vi "Send Value.vi"(8 "error in":errorcluster, 11 "Value":dbl) -> (0 "error out":errorcluster)   [LabVIEW 2014, in "Chart Module.lvlib"]
uses:
  Chart Module.lvlib
  Send Value Argument--cluster.ctl
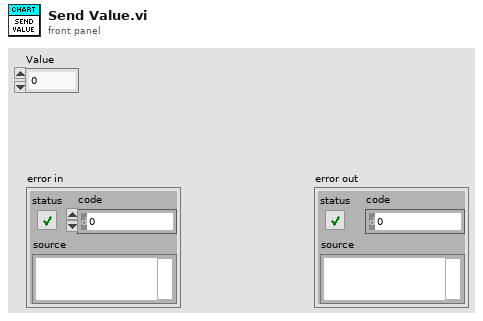
[diagram p1: front panel]
types:
  T1 = typedef "Chart Module.lvlib/Send Value Argument--cluster.ctl" = cluster{"Value":dbl}
  T2 = typedef "Chart Module.lvlib/Request Events--cluster.ctl" = cluster{"Stop Module":refnum<user-event>, "Show Panel":refnum<user-event>, "Hide Panel":refnum<user-event>, "Update Limits":refnum<user-event>, "Send Value":refnum<user-event>, "Clear Chart":refnum<user-event>}
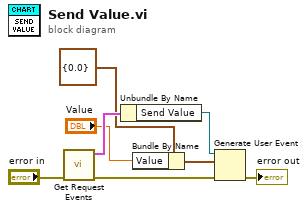
[diagram p0: block diagram]
diagram:
  n1 = call "Get Request Events.vi"("error in"="error in") -> ("error out"=w3:errorcluster, "Request Events"=w8:T2)  [unwired: 9 in]
  n2 = Unbundle By Name(w8) -> ("Send Value"=w7:refnum<user-event>)
  n3 = Bundle By Name(cluster=T1 {"Value"=0.0} ("event data"), "Value"="Value") -> (w4:T1)
  n4 = Generate User Event(user event=w7, event data cluster=w4, error in=w3) -> (error out=→"error out":errorcluster)  [unwired: 1 in, 1 out]
